vi "Core Action.vi"(8 "error in (no error)":errorcluster, 10 "SECS-II Class In":refnum<class "SECS-II Class.lvclass">, 11 "35-CEID EnableDisable in":refnum<class "35-CEID EnableDisable.lvclass">) -> (0 "error out":errorcluster, 2 "SECS-II Class Out":refnum<class "SECS-II Class.lvclass">, 3 "35-CEID EnableDisable out":refnum<class "35-CEID EnableDisable.lvclass">)   [LabVIEW 2020, in "SECS Scenarios.lvlib" / "35-CEID EnableDisable.lvclass"]
uses:
  35-CEID EnableDisable.lvclass
  D:/Dropbox/SECS/SECS_GEM v1.1.0/Com/SECS Scenarios/Scenarios Class/Scenarios Class.lvclass
  SECS Communication/SECS-II Class/SECS-II Class.lvclass
  SECS Communication/S2 Message Class/S2 Message Class.lvclass
  D:/Dropbox/SECS/SECS_GEM v1.1.0/Com/SECS Communication/SECS-II Class/SECS-II Class.lvclass
  Scenarios Class/Reply State.ctl
  Scenarios Class/Scenarios Class.lvclass/Scenarios Class.ctl
  Scenarios Class/Write Reply State.vi
  Scenarios Class/Read HSMS Class.vi
  SECS Communication/HSMS Class/HSMS Class.lvclass
  Scenarios Class/Scenarios Class.lvclass
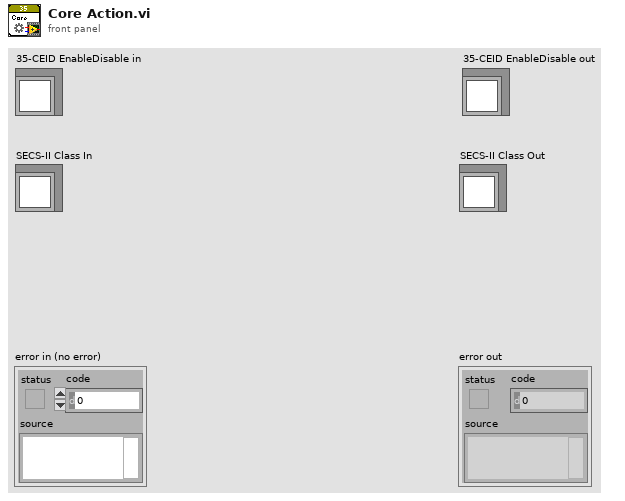
[diagram p1: front panel]
types:
  T1 = typedef "SECS Communication.lvlib/S2 Message Class.lvclass/S2F37.ctl" = cluster{"CEED":bool, "CEID":u32[]}
  T2 = typedef "SECS Scenarios.lvlib/Scenarios Class.lvclass/Reply State.ctl" = enum16{"OK", "Illegal Data", "Unknown Stream", "Unknown Function", "Off-Line", "T3 Timeout", "Inner-Timeout"}
  T3 = typedef "SECS Communication.lvlib/S2 Message Class.lvclass/S2F38.ctl" = enum16{"ok", "denied"}
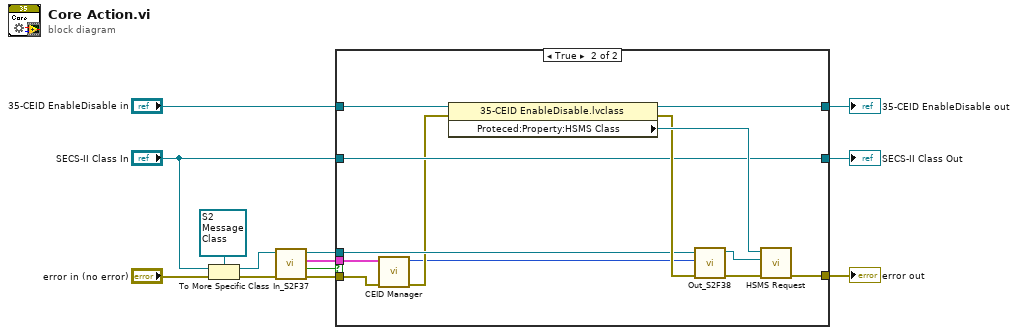
[diagram p0: block diagram]
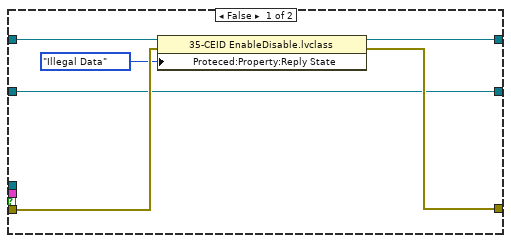
[diagram p2: hidden frame]
diagram:
  n1 = To More Specific Class(target class=refnum<class "S2 Message Class.lvclass"> refnum ("S2 Message Class in"), reference="SECS-II Class In", error in="error in (no error)") -> (specific class reference=w12:refnum<class "S2 Message Class.lvclass">, error out=w13:errorcluster)
  n2 = call "In_S2F37.vi"("error in (no error)"=w13, "S2 Message Class in"=w12) -> ("error out"=w10:errorcluster, "OK?"=w11:bool, "S2F37"=w9:T1, "S2 Message Class out"=w8:refnum<class "S2 Message Class.lvclass">)  [unwired: 6 in]
  n3 = case shown="True" w11 {
    tunnel: w10 -> [w19 w24]
    tunnel: w9 -> [_ w23]
    tunnel: w8 -> [_ w22]
    tunnel: [w17 w31] -> w2
    tunnel: [w16 w30] -> w6
    tunnel: "35-CEID EnableDisable in" -> [w15 w26]
    tunnel: [w14 w25] -> w1
    tunnel: "SECS-II Class In" -> [w14 w25]
    frame False {
      n4 = property class="35-CEID EnableDisable.lvclass"(reference=w15, error in=w19, "Proteced:Property:Reply State"=Reply_State."Illegal Data" ("Reply State")) -> (reference out=w17:refnum<class "35-CEID EnableDisable.lvclass">, error out=w16:errorcluster)
    }
    frame True {
      n5 = call "CEID Manager.vi"("error in (no error)"=w24, "S2F37"=w23) -> ("error out"=w21:errorcluster, "S2F38"=w20:T3)  [unwired: 8 in]
      n6 = property class="35-CEID EnableDisable.lvclass"(reference=w26, error in=w21) -> (reference out=w31:refnum<class "35-CEID EnableDisable.lvclass">, error out=w27:errorcluster, "Proteced:Property:HSMS Class"=w32:refnum<class "HSMS Class.lvclass">)
      n7 = call "Out_S2F38.vi"("error in (no error)"=w27, "S2F38"=w20, "S2 Message Class in"=w22) -> ("error out"=w28:errorcluster, "S2 Message Class out"=w29:refnum<class "S2 Message Class.lvclass">)  [unwired: 7 in]
      n8 = call "HSMS Request.vi"("error in (no error)"=w28, "SECS-II Class In"=w29, "HSMS Class in"=w32) -> ("error out"=w30:errorcluster)  [unwired: 7 in, 1 out]
    }
  }
  "error out" <- w6
  "35-CEID EnableDisable out" <- w2
  "SECS-II Class Out" <- w1
